vi "Vision Processing.vi"(11 "Image In":T1) -> (3 "Height Ratio":dbl)   [LabVIEW 2017]
uses:
  <vilib>/vision/Image Controls.llb/IMAQ Image.ctl
panel:
  out "error out":errorcluster
  out "Border Size":i32=3
  out "Peaks":i32[](array[numeric])
  out "Index Array":i32[](array[numeric])
  out "Waveform Graph":sgl[](graph)
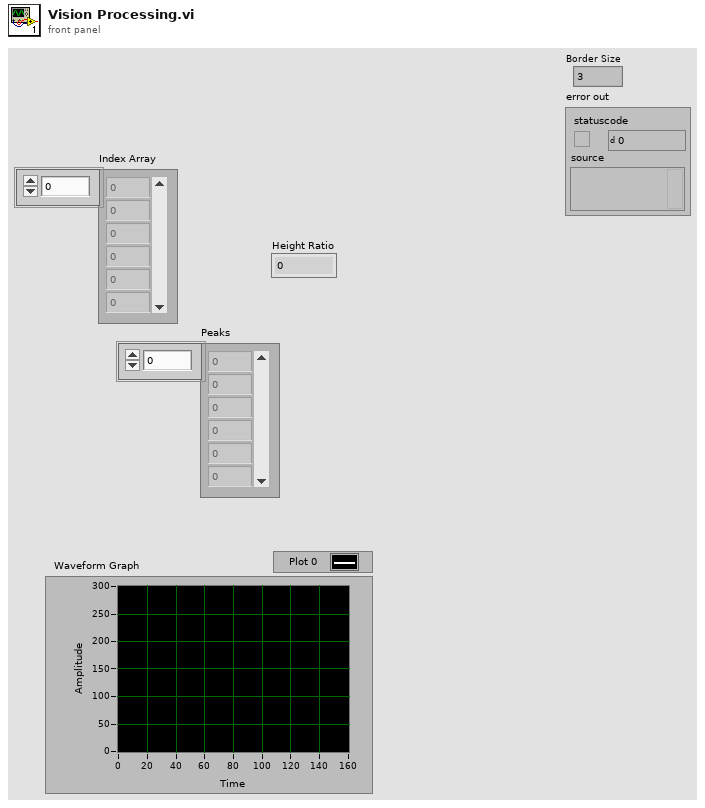
[diagram p1: front panel]
types:
  T1 = typedef "IMAQ Image.ctl" = refnum<image>
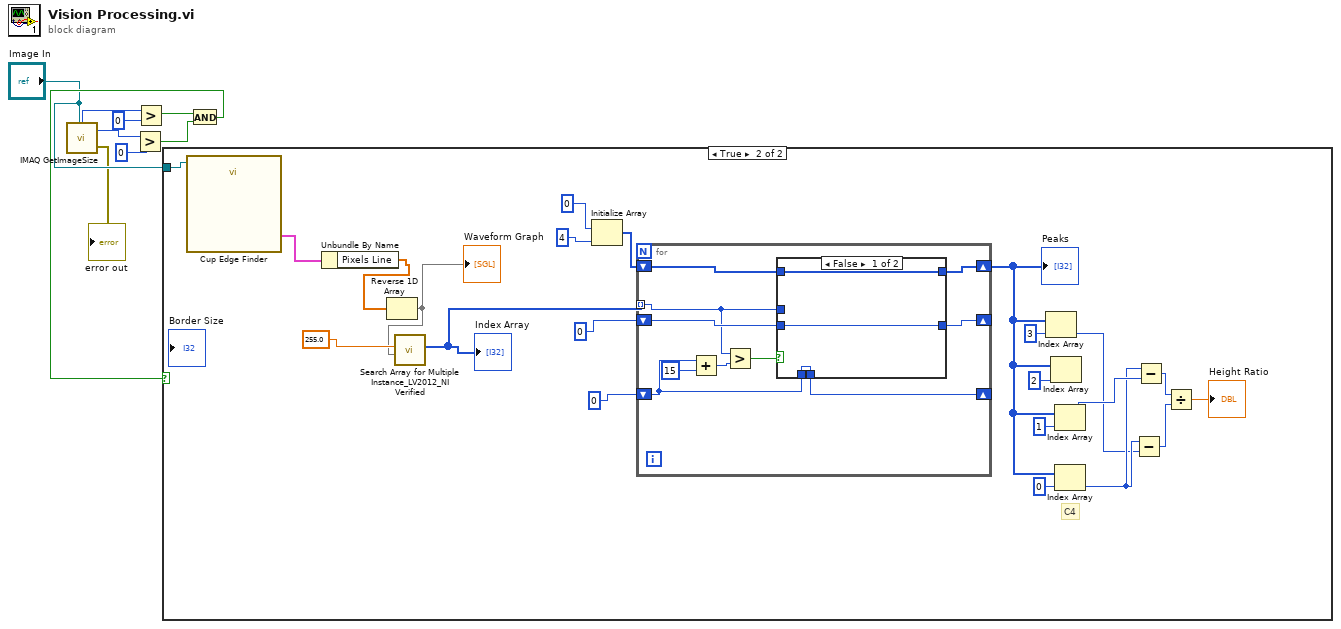
[diagram p0: block diagram]
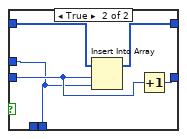
[diagram p3: hidden frame]
diagram:
  n1 = call "IMAQ GetImageSize"("Image"="Image In") -> ("Y Resolution"=w6:i32, "X Resolution"=w9:i32, "error out"=→"error out":errorcluster)  [unwired: 3 in]
  n2 = Greater?(x=w6, y=0) -> (0:w4:bool)
  n3 = Greater?(x=w9, y=0) -> (0:w5:bool)
  n4 = And(x=w5, y=w4) -> (x .and. y?=w3:bool)
  n5 = case shown="True" w3 {
    tunnel: "Image In" -> [_ w12]
    frame False {
    }
    frame True {
      # "C4"
      n6 = call "Cup Edge Finder"("Image In"=w12) -> ("Line Profile (Line Profile 1)"=w22:cluster{"x0":sgl, "dx":sgl, "Pixels Line":sgl[]})  [unwired: 24 in, 2 out]
      n7 = Unbundle By Name(w22) -> ("Pixels Line"=w11:sgl[])
      n8 = Reverse 1D Array(array=w11) -> (reversed array=w10:sgl[])
      "Waveform Graph" <- w10
      n9 = call "Search Array for Multiple Instance_LV2012_NI Verified.vi"("Array to Search"=w10, "Number to find"=255.0) -> ("Index Array"=w23:i32[])  [unwired: 9 in]
      "Index Array" <- w23
      n10 = Initialize Array(0, 4 ("dimension size")) -> (w24:i32[])
      n11 = for {
        tunnel: w23 -> [w35] mode=indexing
        shift-right: [w38] -> _
        shift-left: 0 -> [w39]
        shift-right: [w40] -> w25
        shift-left: w24 -> [w41]
        shift-right: [w37] -> _
        shift-left: 0 -> [w32]
        n12 = Add(x=w32, y=15) -> (x+y=w34:i32)
        n13 = Greater?(x=w35, y=w34) -> (0:w36:bool)
        n14 = case shown="False" w36 {
          tunnel: w41 -> [w44 w49]
          tunnel: [w44 w48] -> w40
          tunnel: w39 -> [w43 w47]
          tunnel: [w43 w46] -> w38
          tunnel: w35 -> [_ w45]
          tunnel: [w42 w45] -> w37
          tunnel: w32 -> [w42 _]
          frame False {
          }
          frame True {
            n15 = Insert Into Array(array=w49, index=w47, new element=w45) -> (w48:i32[])
            n16 = Increment(x=w47) -> (x+1=w46:i32)
          }
        }
      }
      "Peaks" <- w25
      n17 = Index Array(array=w25, index=3) -> (element=w26:i32)
      n18 = Index Array(array=w25, index=2) -> ()  [unwired: 1 out]
      n19 = Index Array(array=w25, index=1) -> (element=w31:i32)
      n20 = Index Array(array=w25, index=0) -> (element=w30:i32)
      n21 = Subtract(x=w30, y=w26) -> (x-y=w28:i32)
      n22 = Subtract(x=w30, y=w31) -> (x-y=w27:i32)
      n23 = Divide(x=w27, y=w28) -> (x/y=→"Height Ratio":dbl)
    }
  }
